vi "Connect.vi"(8 "error in (no error)":errorcluster, 11 "Receiver in":refnum<class "Receiver.lvclass">) -> (0 "error out":errorcluster, 3 "Receiver out":refnum<class "Receiver.lvclass">)   [LabVIEW 2013, in "Receiver.lvlib" / "Receiver.lvclass"]
uses:
  Receiver.lvclass
  Receiver.lvclass/Receiver.ctl
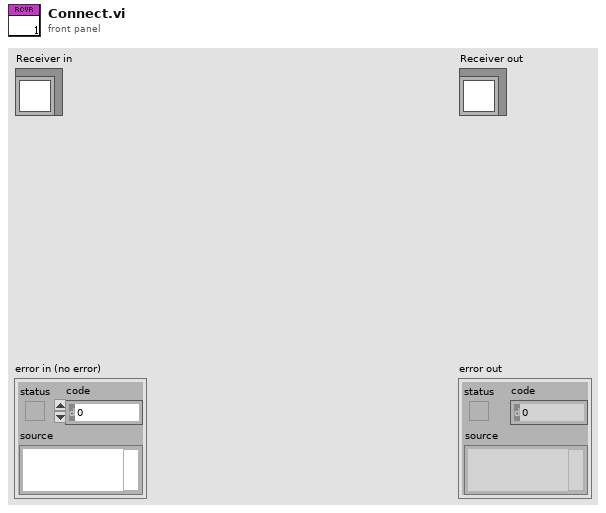
[diagram p1: front panel]
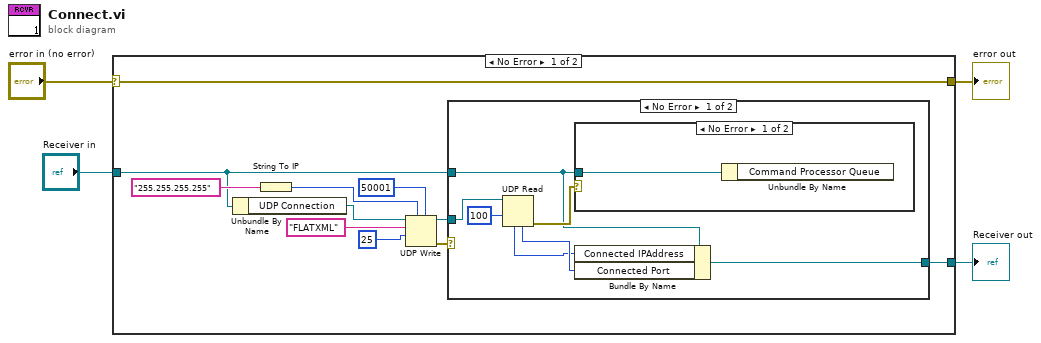
[diagram p0: block diagram]
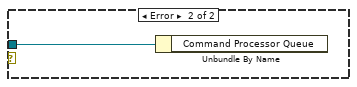
[diagram p2: hidden frame]
diagram:
  n1 = case shown="No Error" "error in (no error)" {
    selector: "error in (no error)" -> [w15 w27]
    tunnel: [w15 w27] -> w3
    tunnel: [w5 w26] -> w1
    tunnel: "Receiver in" -> [w6 w26]
    frame No Error {
      n2 = Unbundle By Name(w6) -> ("UDP Connection"=w14:refnum<k16>)
      n3 = String To IP(1:"255.255.255.255") -> (0:w12:u32)
      n4 = UDP Write(address=w12, port or service name=u16 50001, connection ID=w14, data in="FLATXML", 9:25 ("timeout ms (25000)")) -> (error out=w9:errorcluster, 3:w7:refnum<k16>)  [unwired: 1 in]
      n5 = case shown="No Error" w9 {
        tunnel: w7 -> [w22 _]
        tunnel: w6 -> [w19 w25]
        tunnel: [w18 w25] -> w5
        frame No Error {
          n6 = UDP Read(connection ID=w22, timeout ms (25000)=100) -> (error out=w20:errorcluster, 4:w17:u16, 6:w16:u32)  [unwired: 2 in, 2 out]
          n7 = case "UDP Read Error?" shown="No Error" w20 {
            tunnel: w19 -> [w23 w24]
            frame No Error {
              n8 = Unbundle By Name(w23) -> ()  [unwired: 1 out]
            }
            frame Error {
              n9 = Unbundle By Name(w24) -> ()  [unwired: 1 out]
            }
          }
          n10 = Bundle By Name(cluster=w19, "Connected IPAddress"=w16, "Connected Port"=w17) -> (w18:refnum<class "Receiver.lvclass">)
        }
        frame Error {
        }
      }
    }
    frame Error {
    }
  }
  "error out" <- w3
  "Receiver out" <- w1
